vi "Dashboard Main.vi"() -> ()   [LabVIEW 2017]
uses:
  <vilib>/event_ctls.llb/eventvkey.ctl
  <vilib>/Rock Robotics/WPI/Dashboard/WPI_DashboardLogging Global.vi
  <vilib>/Utility/miscctls.llb/LVRowAndColumnTypeDef.ctl
  <vilib>/Rock Robotics/Network Tables/NT Write Boolean.vi
  <vilib>/Rock Robotics/Network Tables/NT Write Numeric Array.vi
  <vilib>/Rock Robotics/Network Tables/NT Read Numeric Array.vi
  <vilib>/Rock Robotics/Network Tables/NT Read Boolean Array.vi
panel:
  out "error out":errorcluster
  out "error out 2":errorcluster
  in  "Camera Settings Right":T1={"Frame Rate"=30, "Compression"=30, "Size"=1, "DB Camera Config"=FALSE} {"Frame Rate" scale=1.0..30.0; "Compression" scale=100.0..-1.0; "Size" items=["640x480", "320x240", "160x120"]}
  in  "Camera Name Right":string(combo)="No Camera Selection"
  out "Camera Info":cluster{"Mbps LED":bool, "Mbps":dbl, "fps":dbl} {"fps" format="%#.1g"; "Mbps" format="%#.1g"}
  in  "Camera Settings":T1={"Frame Rate"=30, "Compression"=30, "Size"=1, "DB Camera Config"=FALSE} {"Frame Rate" scale=1.0..30.0; "Compression" scale=100.0..-1.0; "Size" items=["640x480", "320x240", "160x120"]}
  in  "TCP":refnum<k5>
  in  "Rec Mode":enum32{"Stop", "Record", "Playback"}(radio)
  out "Robot IP":string
  out "Image Message":string="Timeout in Camera Communications"
  in  "Dashboard Tab":T2(tab)
  out "NT Connection":bool
  out "MotorChart R":cluster{"Numeric":dbl, "Numeric":dbl}(graph)
  out "MotorChart L":cluster{"Numeric":dbl, "Numeric":dbl}(graph)
  out "MotorSliders R":cluster{"MotorSlide1":dbl, "MotorSlide2":dbl} {"MotorSlide2" scale=-1.0..1.0 scale format="%#_2e"; "MotorSlide1" scale=-1.0..1.0 scale format="%#_2e"}
  out "MotorSliders L":cluster{"MotorSlide1":dbl, "MotorSlide2":dbl} {"MotorSlide2" scale=-1.0..1.0 scale format="%#_2e"; "MotorSlide1" scale=-1.0..1.0 scale format="%#_2e"}
  out "JS1 Z":dbl(slide) scale=-1.0..1.0 scale format="%#_2e"
  out "JS1 Graph":cluster{"X":dbl, "Y":dbl}[](graph)
  out "JS1 Buttons":T3
  out "JS2 Z":dbl(slide) scale=-1.0..1.0 scale format="%#_2e"
  out "JS2 Graph":cluster{"X":dbl, "Y":dbl}[](graph)
  out "JS2 Buttons":T3
  out "Mode":T4(ring)=enum."Auto Disabled"
  out "Gear State":string="Waiting...."
  out "Camera Image Right":T5(plugin-control)
  in  "Ring":u16(ring)
  in  "Select Robot Position":string(combo)="Select Robot Position ..."
  in  "Select Auto":string(combo)="Select Autonomous ..."
  in  "Left String":string
  in  "Right String":string
  in  "Save Left Auto":bool
  in  "Load Left Auto":bool
  in  "Save Right Auto":bool
  in  "Load Right Auto":bool
  out "new picture":picture
  in  "Starting Pos":i16(slide)=128 scale=340.0..50.0
  in  "Test Slider":dbl(slide) scale=0.0..100.0 scale format="%#_3g"
  in  "On/Off":bool caption="Solenoid"
  in  "Test Name":u16(ring) items=["Select the test to run..."]
  in  "Test Tree":string(tree)
  in  "Motor":cluster{"Value":dbl, "Enable":bool} {"Value" scale=-1.0..1.0 scale format="%#_3g"}
  out "Progress":T6 {"Test Progress" scale=0.0..100.0}
  in  "Rev/Fwd":cluster{"Forward":bool, "Reverse":bool}
  in  "Test Ring":u16(ring) items=["Monochrome", "Color"]
  out "Cmd Status":string
  in  "Execute Command":bool
  in  "Command Params":string[][](table)
  in  "Command Selection":i32(listbox)
  in  "CheckList":i32(listbox)
  out "Tree":string(tree)
  in  "Key Binds":u16[](array[ring]) items=["No Function", "Gear Shift", "Direction Toggle", "Cube Up", "Cube Down", "LRamp Deploy", "RRamp Deploy", "LRamp Raise", "RRamp Raise"]
  in  "High Gear":bool=TRUE
  in  "Direction Toggle":bool=TRUE
  in  "Autoshift":bool=TRUE
  in  "Max Speed":dbl=1.0 format="%#_13g"
  in  "Foreward Deadzone":dbl=1.0 format="%#_13g"
  in  "Turning Deadzone":dbl=0.4 format="%#_13g"
  in  "High Gear Turning Multiplier":dbl=0.65 format="%#_13g"
  in  "Save":bool
  in  "Load":bool
  out "Profile Name":string="Profile1"
  in  "Control System":T7(ring)
  in  "Turning Multiplier":dbl=1.0 format="%#_13g"
  out "Boolean Array":bool[](array[boolean])
  out "Time":dbl
  in  "Points Speed":dbl[][](array[slide]) scale=0.0..1.0
  out "Speed Graph":cluster{dbl[], dbl[]}[](graph)
  in  "Points Turning":dbl[][](array[slide]) scale=0.0..1.0
  out "Turning Graph":cluster{dbl[], dbl[]}[](graph)
  out "Camera Image":T5(plugin-control)
  out "Background":bool
  in  "Camera Name":string(combo)="No Camera Selection"
  # "HW"
  # "HW"
  # "Joysticks"
  # "Drive Motors"
  # "Front"
  # "Right"
  # "Left"
  # "Back"
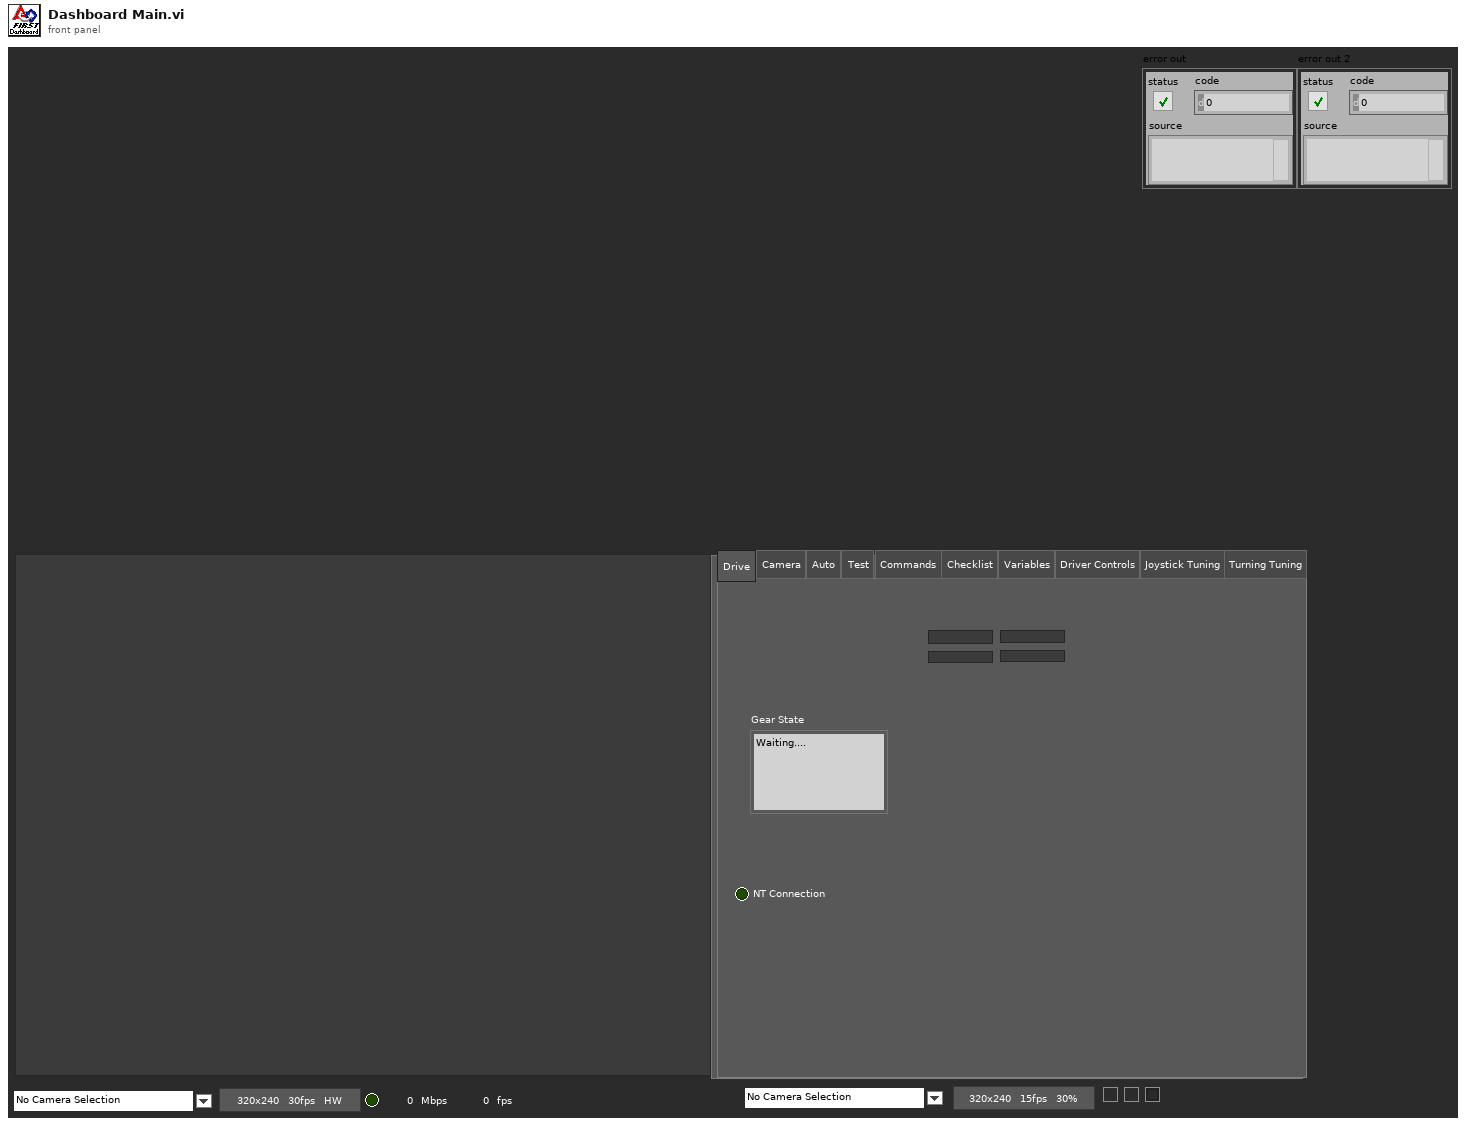
[diagram p1: front panel]
types:
  T1 = cluster{"Frame Rate":i32, "Compression":i32, "Size":u16, "DB Camera Config":bool}
  T2 = enum32{"Drive", "Camera", "Basic", "Auto", "Test", "Commands", "Checklist", "Variables", "Driver Controls", "Joystick Tuning", "Turning Tuning"}
  T3 = cluster{bool, bool, bool, bool, bool, bool, bool, bool, bool, bool, bool, bool}
  T4 = enum8{"Tele-Op Disabled", "Tele-Op Enabled", "Auto Disabled", "Auto Enabled", "Test Disabled", "Test Enabled", "Disconnected", "No Code", "E-Stop"}
  T5 = typedef "IMAQ Image.ctl" = refnum<image>
  T6 = cluster{"Test Progress":u8, "Test Progress Text":string}
  T7 = enum16{"Arcade Drive", "Two Part Arcade Drive", "Tank"}
  T8 = cluster{"Save Path":path, "Interval (s)":dbl, "Keep":i32}
  T9 = enum32{"Drive", "Camera", "Basic", "Custom", "Test", "Commands", "Checklist", "Variables"}
  T10 = typedef "Image Type" = u32
  T11 = cluster{"IDs":cluster{"RPC field ID":u16, "Unique ID":u16}, "String":string}
  T12 = enum32{"Drive", "Camera", "Basic", "Auto", "Test", "Commands", "Checklist", "Variables"}
  T13 = cluster{"Error Strings":string, "Disable Counts":cluster{u16, u16}, "Rail Faults":cluster{u16, u16, u16}, "Robot IP":string, "DB Mode":u8, "Event Info":cluster{"Name":string, "Type":u8, "Number":u16, "Replay":u8}}
  T14 = cluster{"Storage":cluster{"Disk Free":u64, "RAM Block":u32, "RAM free":u32}, "CPU Utilization":cluster{"CPU % ISR":sgl, "CPU % Time Crit":sgl, "CPU % Timed Str":sgl, "CPU % High":sgl, "CPU % Above":sgl, "CPU % Normal":sgl, "CPU % Low":sgl}, "CAN":cluster{"% Bus Utilization":sgl, "Bus Off Cnt":u32, "TX_FIFO Full Cnt":u32, "Receive Error Cnt":u8, "Transmit Error Cnt":u8}, "HID":cluster{"HID Outputs":u32, "Rumble Low":u16, "Rumble High":u16}[]}
  T15 = cluster{"Status bits":cluster{"Test Mode":bool, "Autonomous":bool, "Enabled":bool, "Code Start":bool, "Brownout":bool, "Reserved 2":bool, "Reserved 3":bool, "E-Stop":bool}, "Code Trace":cluster{"Disabled":bool, "TeleOp":bool, "Auto":bool, "Test":bool}, "Controller Type":enum16{"unknown", "cRIO", "roboRio"}, "Code?":enum16{"unknown", "noCode", "code"}, "Battery V":dbl}
  T16 = cluster{"Control Bits":cluster{"TestMode":bool, "Autonomous":bool, "Enabled":bool, "FMS Present":bool, bool, bool, bool, "E-Stop":bool}, "Team Station ":u8, "Countdown":sgl, "Joystick Values":cluster{"Axes":dbl[], "Buttons":bool[], "POVs":i16[]}[]}
  T17 = cluster{"Axes":dbl[], "Buttons":bool[], "POVs":i16[]}[]
  T18 = cluster{"Axes":dbl[], "Buttons":bool[], "POVs":i16[]}
  T19 = cluster{"Buttons[0]":bool, "Buttons[1]":bool, "Buttons[2]":bool, "Buttons[3]":bool, "Buttons[4]":bool, "Buttons[5]":bool, "Buttons[6]":bool, "Buttons[7]":bool, "Buttons[8]":bool, "Buttons[9]":bool, "Buttons[10]":bool, "Buttons[11]":bool}
  T20 = cluster{"High Gear Turning Multiplier":refnum<vi>, "Turning Deadzone":refnum<vi>, "Foreward Deadzone":refnum<vi>, "Max Speed":refnum<vi>, "Autoshift":refnum<vi>, "High Gear":refnum<vi>, "Direction Toggle":refnum<vi>, "Control System":refnum<vi>, "Turning Multiplier":refnum<vi>, "Profile Name":refnum<vi>, "Key Binds":refnum<vi>}
  T21 = cluster{"Camera Image":refnum<vi>, "Dashboard Tab":refnum<vi>, "Background":refnum<vi>, "Rec Mode":refnum<vi>, "Test Slider":refnum<vi>, "On/Off ":refnum<vi>, "Test Ring":refnum<vi>, "Rev/Fwd":refnum<vi>, "Test Name":refnum<vi>, "Motor":refnum<vi>, "Progress":refnum<vi>, "CheckList":refnum<vi>, "Tree":refnum<vi>, "Test Tree":refnum<vi>, "Command Params":refnum<vi>, "Command Selection":refnum<vi>, "Execute Command":refnum<vi>, "Cmd Status":refnum<vi>, "Camera Settings":refnum<vi>, "Camera Name":refnum<vi>, "Camera Info":refnum<vi>, "Camera Settings Right":refnum<vi>, "Camera Name Right":refnum<vi>, "Camera Image Right":refnum<vi>}
  T22 = cluster{"Camera Name Right":string, string, "Saved DB Images Info":cluster{"Save Path":path, "Interval (s)":dbl, "Keep":i32}}
  T23 = cluster{"Camera Name":string, string, "Saved DB Images Info":cluster{"Save Path":path, "Interval (s)":dbl, "Keep":i32}}
  T24 = cluster{"Operation":enum16{"Update", "Clear"}, "Color Box":u32}[]
  T25 = typedef "eventvkey.ctl" = enum16{"ASCII", "Enter", "Return", "Shift", "Ctrl", "Alt", "Cmd", "Opt", "Caps", "NumLock", "Clear", "Break", "Up", "Down", "Left", "Right", "Insert", "Delete", "Home", "End", "PageUp", "PageDown", "Escape", "Help", "Pause", "ScrollLock", "F1", "F2", "F3", "F4", "F5", "F6", "F7", "F8", "F9", "F10", "F11", "F12", "F13", "F14", "F15", "F16", "F17", "F18", "F19", "F20", "F21", "F22", "F23", "F24", "Play", "VolumeUp", "VolumeDown", "Mute", "Two Byte Char"}
  T26 = cluster{"Image Size":bool, "Image Type":bool, "Pixel Value":bool, "ROI Information":bool, "Zoom Factor":bool}
  T27 = cluster{"Operation":enum16{"Update", "Clear"}, "Color Box":u32}
  T28 = typedef "LVRowAndColumnTypeDef.ctl" = cluster{"Row":i32, "Column":i32}
  T29 = cluster{"Shift":bool, "Ctrl":bool, "Alt":bool, "Cmd":bool, "Opt":bool}
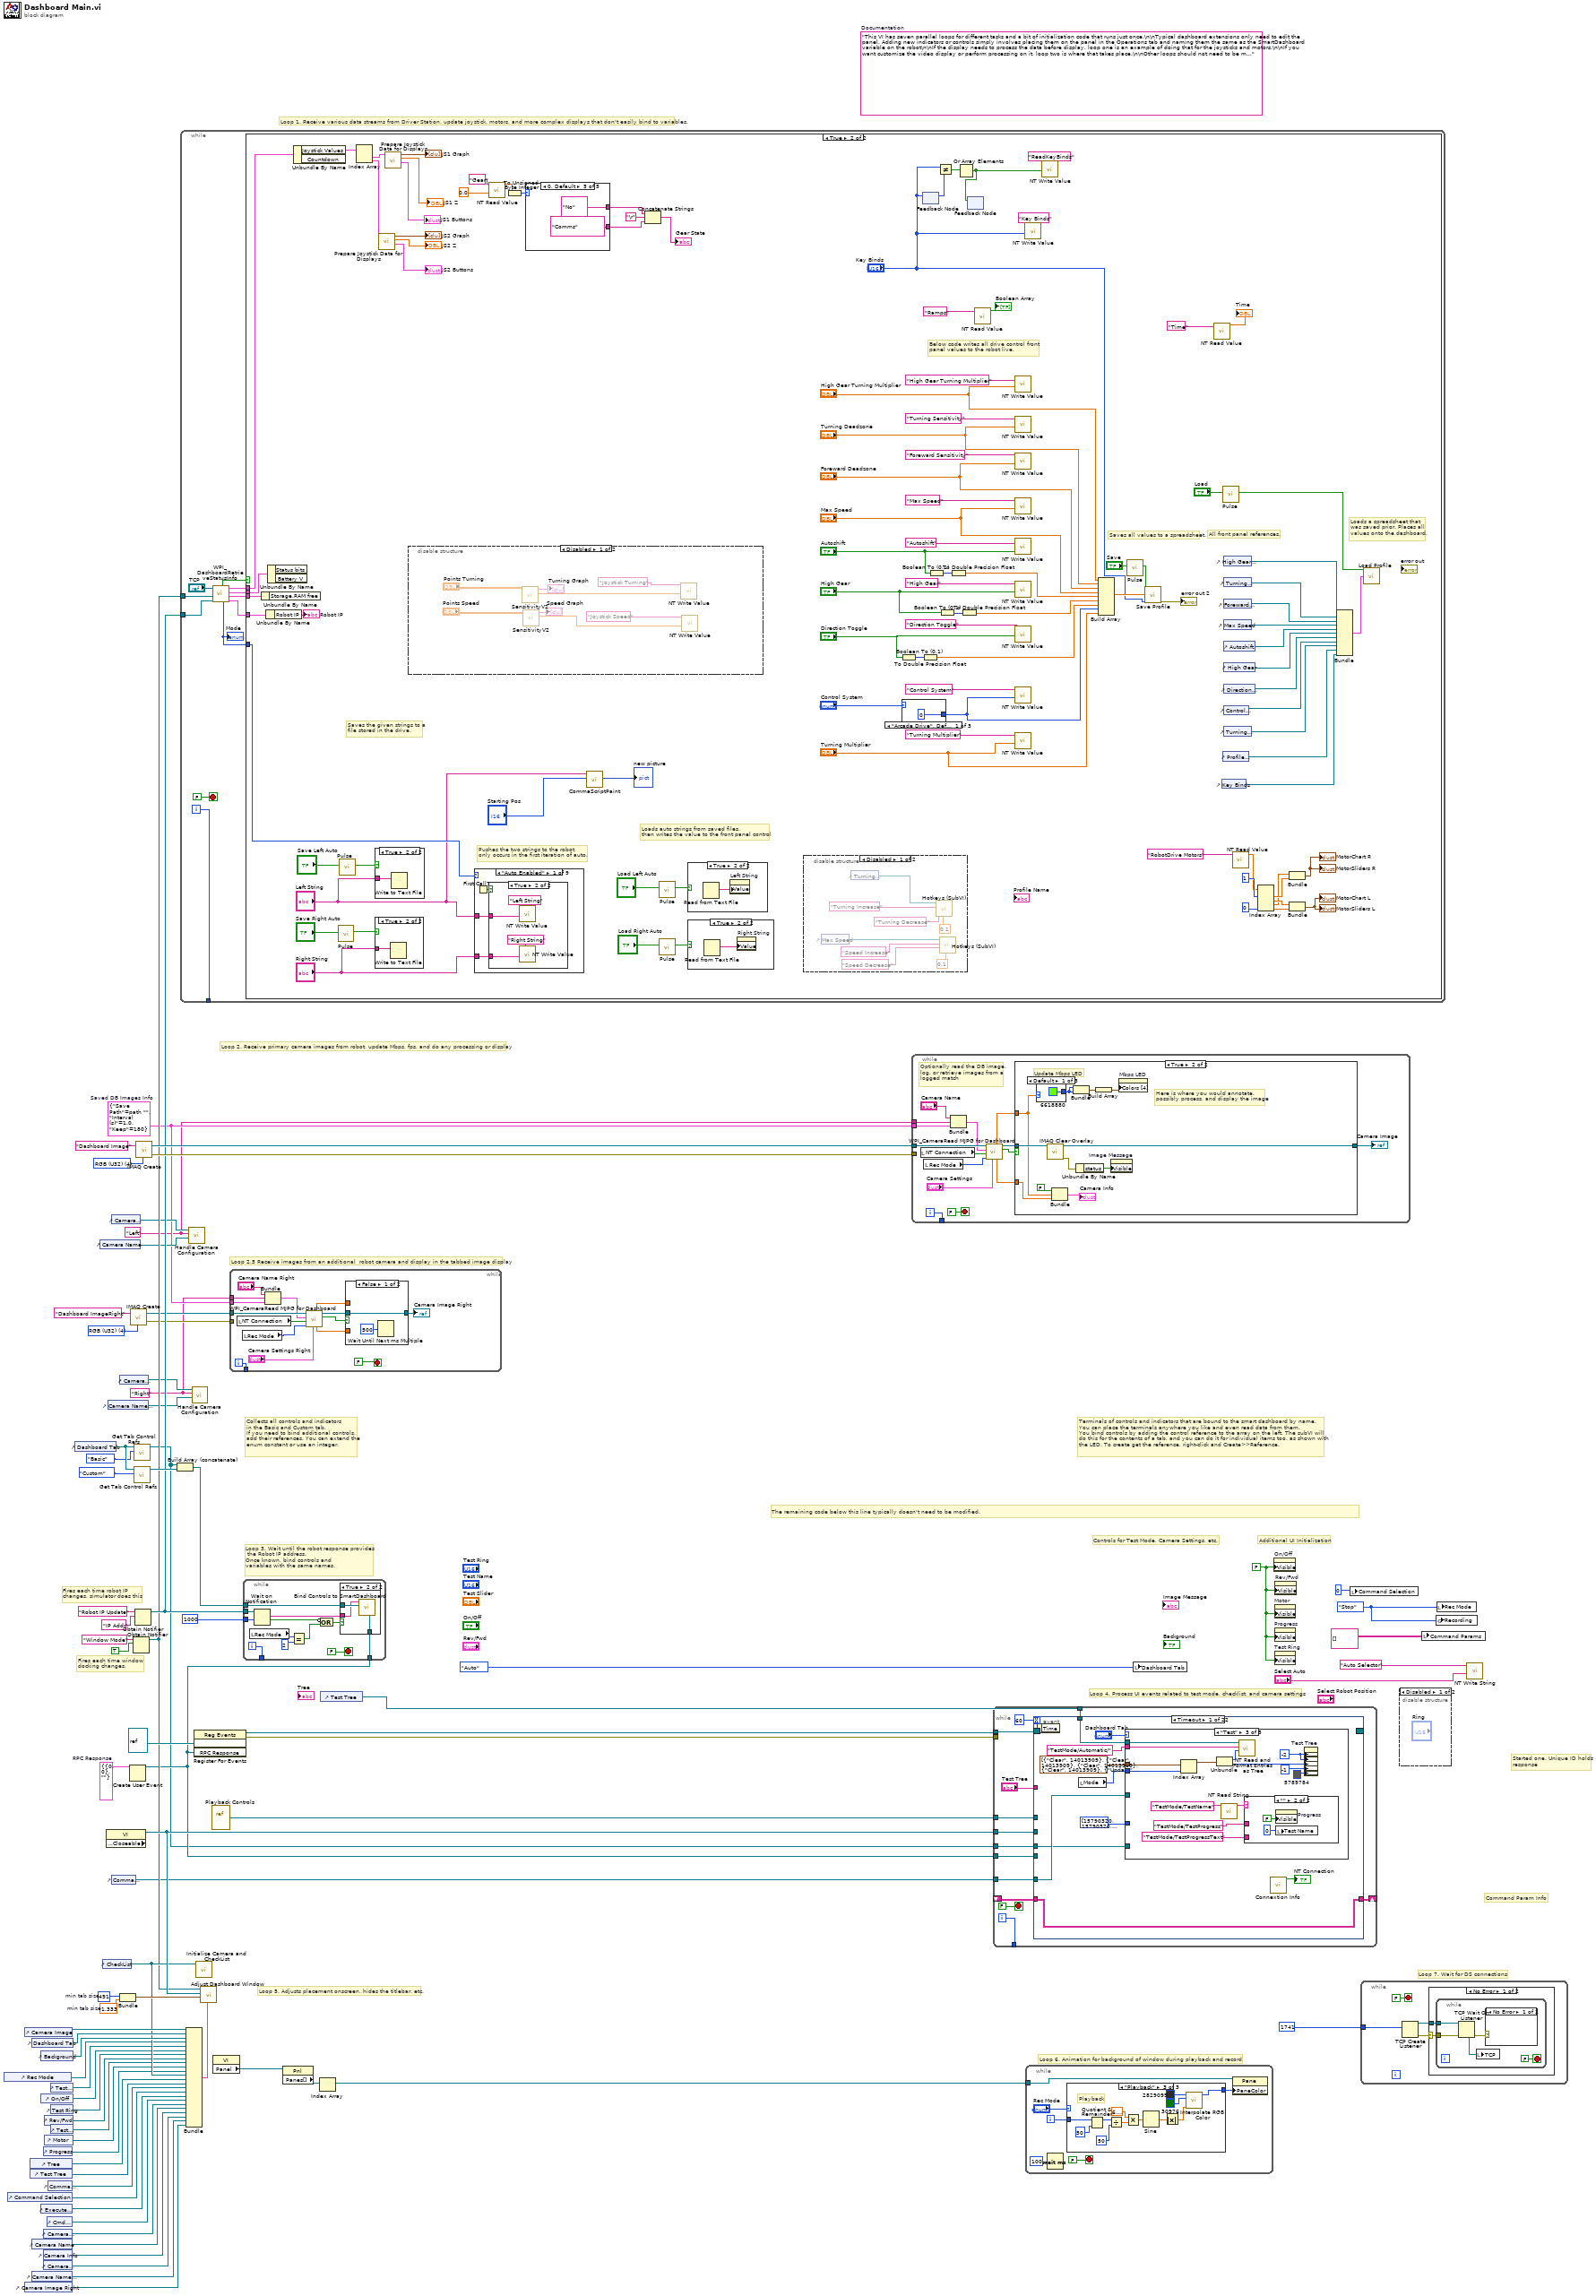
[diagram p0: block diagram]
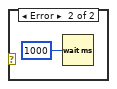
[diagram p4: hidden frame]
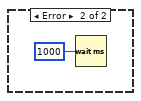
[diagram p5: hidden frame]
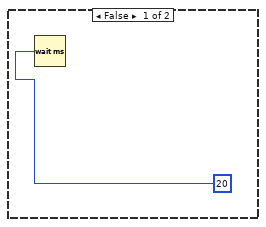
[diagram p6: hidden frame]
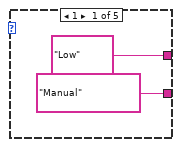
[diagram p8: hidden frame]
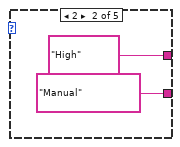
[diagram p9: hidden frame]
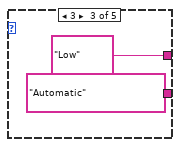
[diagram p10: hidden frame]
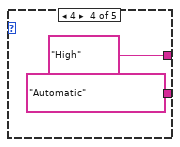
[diagram p11: hidden frame]
diagram:
  w4 = T8 {"Save Path"=path "", "Interval (s)"=1.0, "Keep"=180}  # Saved DB Images Info
  w3 = "Right"
  w2 = "Left"
  w14 = T10 4 items=["Grayscale (U8)", "Grayscale (I16)", "Grayscale (SGL)", "Complex (CSG)", "RGB (U32)", "HSL (U32)", "RGB (U64)"] ("Image Type")
  w29 = T11 {"IDs"={"RPC field ID"=0, "Unique ID"=0}, "String"=""}  # RPC Response
  w52 = 491  # min tab size
  w51 = 1.333  # min tab size
  w59 = enum32{"Stop", "Record", "Playback"}."Stop" ("Rec Mode")
  w36 = FALSE ("Visible")
  (unwired) "This VI has seven parallel loops for different tasks and a bit of initialization code that runs just once.\n\nTypical dashboard extensions only need to edit the panel. Adding new indicators or controls simply involves placing them on the panel in the Operations tab and naming them the same as the SmartDashboard variable on the robot\n\nIf the display needs to process the data before display, loop one is an example of doing that for the joysticks and motors.\n\nIf you want customize the video display or perform processing on it, loop two is where that takes place.\n\nOther loops should not need to be modified. They are pretty standard, and document the task they perform."  # Documentation
  w76 = T10 4 items=["Grayscale (U8)", "Grayscale (I16)", "Grayscale (SGL)", "Complex (CSG)", "RGB (U32)", "HSL (U32)", "RGB (U64)"] ("Image Type")
  # "Loop 2.5 Receive images from an additional  robot camera and display in the tabbed image display"
  # "Command Param Info"
  # "Started one, Unique ID holds\nresponse"
  # "Loop 7. Wait for DS connections"
  # "Controls for Test Mode, Camera Settings, etc."
  # "Additional UI Initialization"
  # "Loop 6. Animation for background of window during playback and record"
  # "Fires each time robot IP\nchanges, simulator does this"
  # "Fires each time window\ndocking changes."
  # "Collects all controls and indicators\nin the Basic and Custom tab.\nIf you need to bind additional controls,\nadd their references. You can extend the\nenum constant or use an integer."
  # "The remaining code below this line typically doesn't need to be modified."
  # "Loop 4. Process UI events related to test mode, checklist, and camera settings"
  # "Terminals of controls and indicators that are bound to the smart dashboard by name.\nYou can place the terminals anywhere you like and even read data from them.\nYou bind controls by adding the control reference to the array on the left. The subVI will\ndo this for the contents of a tab, and you can do it for individual items too, as shown with\nthe LED. To create get the reference, right-click and Create>>Reference."
  # "Loop 3. Wait until the robot response provides\n the Robot IP address.\nOnce known, bind controls and\nvariables with the same names."
  # "Loop 5. Adjusts placement onscreen, hides the titlebar, etc."
  # "Loop 1. Receive various data streams from Driver Station, update joystick, motors, and more complex displays that don't easily bind to variables."
  # "Loop 2. Receive primary camera images from robot, update Mbps, fps, and do any processing or display"
  n1 = control-ref of="Rec Mode"() -> (w42:refnum<vi>)
  n2 = control-ref of="Command Selection"() -> (w28:refnum<vi>)
  n3 = control-ref of="Camera Image Right"() -> (w7:refnum<vi>)
  n4 = control-ref of="Camera Image"() -> (w54:refnum<vi>)
  n5 = control-ref of="Tree"() -> (w46:refnum<vi>)
  n6 = control-ref of="Test Tree"() -> (w45:refnum<vi>)
  n7 = control-ref of="Dashboard Tab"() -> (w53:refnum<vi>)
  n8 = control-ref of="Camera Name"() -> (w19:refnum<vi>)
  n9 = control-ref of="Camera Name Right"() -> (w8:refnum<vi>)
  n10 = control-ref of="Execute Command"() -> (w30:refnum<vi>)
  n11 = control-ref of="Background"() -> (w49:refnum<vi>)
  n12 = control-ref of="On/Off"() -> (w40:refnum<vi>)
  n13 = control-ref of="Progress"() -> (w37:refnum<vi>)
  n14 = control-ref of="Camera Settings"() -> (w20:refnum<vi>)
  n15 = control-ref of="Camera Info"() -> (w18:refnum<vi>)
  n16 = control-ref of="Camera Settings Right"() -> (w9:refnum<vi>)
  n17 = control-ref of="Rev/Fwd"() -> (w38:refnum<vi>)
  n18 = control-ref of="Motor"() -> (w43:refnum<vi>)
  n19 = control-ref of="Cmd Status"() -> (w24:refnum<vi>)
  n20 = control-ref of="Command Params"() -> (w31:refnum<vi>)
  n21 = control-ref of="Test Slider"() -> (w41:refnum<vi>)
  n22 = control-ref of="Test Ring"() -> (w39:refnum<vi>)
  n23 = control-ref of="Test Name"() -> (w44:refnum<vi>)
  n24 = control-ref of="Dashboard Tab"() -> (w57:refnum<vi>)
  n25 = control-ref of="Camera Name"() -> (w21:refnum<vi>)
  n26 = control-ref of="CheckList"() -> (w47:refnum<vi>)
  n27 = property class="VI" props=["Front Panel.Closeable"]() -> (reference out=w58:refnum<vi>)  [unwired: 2 in, 2 out]
  n28 = control-ref of="Camera Name Right"() -> (w10:refnum<vi>)
  n29 = control-ref of="Camera Settings"() -> (w22:refnum<vi>)
  n30 = control-ref of="Command Params"() -> (w23:refnum<vi>)
  n31 = control-ref of="Camera Settings Right"() -> (w11:refnum<vi>)
  n32 = Bundle("min tab size"=w52, "min tab size"=w51) -> (w50:cluster{"min tab size":i32, "min tab size":dbl})  [unwired: 1 in]
  n33 = Create User Event(user event datatype=w29) -> (user event=w25:refnum<user-event>)  [unwired: 1 in, 1 out]
  n34 = call "IMAQ Create"("Image Name"="Dashboard ImageRight", "Image Type"=w14) -> ("New Image"=w13:T5, "error out"=w12:errorcluster)  [unwired: 2 in, 1 out]
  n35 = Obtain Notifier(name (unnamed)="Window Mode", notification data type=TRUE) -> (notifier out=w34:refnum<notifier>)  [unwired: 2 in, 2 out]
  n36 = call <vilib>:"Get Tab Control Refs.vi"("Page Index"=T9."Basic" ("Dashboard Tab"), "TabControl in"=w57) -> ("ControlsOnPage"=w17:refnum<vi>[])  [unwired: 9 in]
  n37 = call <vilib>:"Get Tab Control Refs.vi"("Page Index"=T9."Custom" ("Dashboard Tab"), "TabControl in"=w57) -> ("ControlsOnPage"=w56:refnum<vi>[])  [unwired: 9 in]
  n38 = Obtain Notifier(name (unnamed)="Robot IP Update", notification data type="IP Addr" ("name (unnamed)")) -> (notifier out=w35:refnum<notifier>)  [unwired: 2 in, 2 out]
  n39 = call "IMAQ Create"("Image Name"="Dashboard Image", "Image Type"=w76) -> ("New Image"=w74:T5, "error out"=w73:errorcluster)  [unwired: 2 in, 1 out]
  n40 = Build Array (concatenate)(w17, w56) -> (w55:refnum<vi>[])
  n41 = while {
    tunnel: [w86] -> _
    tunnel: w35 -> [w80]
    tunnel: w34 -> [w77]
    i -> [w86]
    stop <- FALSE stop-if-true
    n42 = call <vilib>:"WPI_DashboardRetrieveStatusInfo.vi"("Binding Refnum"=w80, "Window Mode Notifier"=w77, "TCP Cnx"="TCP") -> ("Power and Errors"=w81:T13, "Robot Metrics"=w84:T14, "Status Info"=w85:T15, "Control Info"=w82:T16, "Robot Mode"=w79:T4, "Process?"=w83:bool)  [unwired: 3 in]
    "Mode" <- w79
    n43 = case shown="True" w83 {
      tunnel: w85 -> [_ w186]
      tunnel: w84 -> [_ w185]
      tunnel: w82 -> [_ w184]
      tunnel: w81 -> [_ w183]
      tunnel: w79 -> [_ w113]
      frame False {
        n44 = Wait (ms)(milliseconds to wait=u32 20) -> ()  [unwired: 1 out]
      }
      frame True {
        # "Loads a spreadsheet that\nwas saved prior. Places all\nvalues onto the dashboard."
        # "All front panel references."
        # "Saves all values to a spreadsheet."
        # "Below code writes all drive control front\npanel values to the robot live."
        # "Pushes the two strings to the robot,\nonly occurs in the first iteration of auto."
        # "Saves the given strings to a\nfile stored in the drive."
        # "Loads auto strings from saved files,\nthen writes the value to the front panel control"
        n45 = Unbundle By Name(w185) -> ()  [unwired: 1 out]
        n46 = Unbundle By Name(w183) -> ("Robot IP"=→"Robot IP":string)
        n47 = Unbundle By Name(w186) -> ()  [unwired: 2 out]
        n48 = Unbundle By Name(w184) -> ("Joystick Values"=w174:T17)  [unwired: 1 out]
        n49 = call "Pulse.vi"("Input"="Save Right Auto") -> ("Output"=w117:bool)  [unwired: 10 in]
        n50 = call "Pulse.vi"("Input"="Save Left Auto") -> ("Output"=w121:bool)  [unwired: 10 in]
        n51 = Index Array(array=w174) -> (element #1=w173:T18, element #2=w169:T18)  [unwired: 2 in]
        n52 = case shown="True" w117 {
          tunnel: "Right String" -> [_ w220]
          frame False {
          }
          frame True {
            n53 = Write to Text File(text=w220) -> ()  [unwired: 3 in, 3 out]
          }
        }
        n54 = case shown="True" w121 {
          tunnel: "Left String" -> [_ w223]
          frame False {
          }
          frame True {
            n55 = Write to Text File(text=w223) -> ()  [unwired: 3 in, 3 out]
          }
        }
        n56 = call "Prepare Joystick Data for Displays.vi"("Joystick Values"=w169) -> ("Buttons"=→"JS2 Buttons":T19, "Z Axis"=→"JS2 Z":dbl, "Cartesian Data"=→"JS2 Graph":cluster{"X axis":dbl, "X axis":dbl}[])  [unwired: 8 in]
        n57 = call "Prepare Joystick Data for Displays.vi"("Joystick Values"=w173) -> ("Buttons"=→"JS1 Buttons":T19, "Z Axis"=→"JS1 Z":dbl, "Cartesian Data"=→"JS1 Graph":cluster{"X axis":dbl, "X axis":dbl}[])  [unwired: 8 in]
        n58 = disable-structure shown="Disabled" {
          frame Disabled {
            n59 = call "SensitivityV2.vi"("Points"="Points Turning") -> ("Yi"=w187:dbl[], "XY Graph"=→"Turning Graph":cluster{dbl[], dbl[]}[])  [unwired: 9 in]
            n60 = call "SensitivityV2.vi"("Points"="Points Speed") -> ("Yi"=w190:dbl[], "XY Graph"=→"Speed Graph":cluster{dbl[], dbl[]}[])  [unwired: 9 in]
            n61 = call-poly <vilib>:"NT Write Value.vi"("Numeric Array"=w187, "Name"="Joystick Turning") -> ()  [unwired: 9 in, 1 out]
            n62 = call-poly <vilib>:"NT Write Value.vi"("Numeric Array"=w190, "Name"="Joystick Speed") -> ()  [unwired: 9 in, 1 out]
          }
          frame Enabled {
          }
        }
        n63 = case shown="\"Auto Enabled\"" w113 {
          tunnel: "Left String" -> [w215 _ _ _ _ _ _ _ _]
          tunnel: "Right String" -> [w214 _ _ _ _ _ _ _ _]
          frame "Auto Enabled" {
            n64 = First Call?() -> (First Call?: T/F=w213:bool)
            n65 = case shown="True" w213 {
              tunnel: w215 -> [_ w219]
              tunnel: w214 -> [_ w218]
              frame False {
              }
              frame True {
                n66 = call-poly <vilib>:"NT Write Value.vi"("String"=w219, "Name"="Left String") -> ()  [unwired: 9 in, 1 out]
                n67 = call-poly <vilib>:"NT Write Value.vi"("String"=w218, "Name"="Right String") -> ()  [unwired: 9 in, 1 out]
              }
            }
          }
          frame "Test Disabled" {
          }
          frame "Test Enabled" {
          }
          frame "Disconnected" {
          }
          frame "No Code" {
          }
          frame "E-Stop" {
          }
          frame "Auto Disabled" {
          }
          frame "Tele-Op Enabled" {
          }
          frame "Tele-Op Disabled" {
          }
        }
        n68 = call-poly <vilib>:"NT Read Value.vi"("Default Value"=0.0, "Name"="Gear") -> ("Numeric"=w106:dbl)  [unwired: 8 in, 1 out]
        n69 = To Unsigned Byte Integer(number=w106) -> (unsigned 8bit integer=w105:u8)
        n70 = case shown="0, Default" w105 {
          tunnel: ["Low" "High" "Low" "High" "No"] -> w109
          tunnel: ["Manual" "Manual" "Automatic" "Automatic" "Comms"] -> w111
          frame 1 {
          }
          frame 2 {
          }
          frame 3 {
          }
          frame 4 {
          }
          frame 0, Default {
          }
        }
        n71 = call "CommaScriptPaint.vi"("string 2"="Starting Pos", "string"="Left String") -> ("new picture"=→"new picture":picture)  [unwired: 8 in, 1 out]
        n72 = Concatenate Strings(w109, "\r", w111) -> (→"Gear State":string)
        n73 = call "Pulse.vi"("Input"="Load Left Auto") -> ("Output"=w120:bool)  [unwired: 10 in]
        n74 = call "Pulse.vi"("Input"="Load Right Auto") -> ("Output"=w114:bool)  [unwired: 10 in]
        n75 = case shown="True" w120 {
          frame False {
          }
          frame True {
            n76 = Read from Text File() -> (text=w222:string)  [unwired: 4 in, 3 out]
            n77 = property on="Left String" class="Str"("Value"=w222) -> ()  [unwired: 2 in, 2 out]
          }
        }
        n78 = case shown="True" w114 {
          frame False {
          }
          frame True {
            n79 = Read from Text File() -> (text=w221:string)  [unwired: 4 in, 3 out]
            n80 = property on="Right String" class="Str"("Value"=w221) -> ()  [unwired: 2 in, 2 out]
          }
        }
        n81 = disable-structure shown="Disabled" {
          frame Disabled {
            n82 = control-ref of="Max Speed"() -> (w209:refnum<vi>)
            n83 = control-ref of="Turning Multiplier"() -> (w212:refnum<vi>)
            n84 = call "Hotkeys (SubVI).vi"("Iteration Quantity"=0.1, "Decrease"="Turning Decrease", "Increase"="Turning Increase", "Reference"=w212) -> ()  [unwired: 8 in]
            n85 = call "Hotkeys (SubVI).vi"("Iteration Quantity"=0.1, "Decrease"="Speed Decrease", "Increase"="Speed Increase", "Reference"=w209) -> ()  [unwired: 8 in]
          }
          frame Enabled {
          }
        }
        n86 = Boolean To (0,1)(Boolean="Direction Toggle") -> (0, 1=w145:i16)
        n87 = case shown="\"Arcade Drive\", Default" "Control System" {
          tunnel: [0 1 2] -> w122
          frame "Arcade Drive", Default {
          }
          frame "Two Part Arcade Drive" {
          }
          frame "Tank" {
          }
        }
        n88 = feedback-in #1("Key Binds") -> ()
        n89 = feedback #1() -> (w104:u16[])  [unwired: 1 in]
        n90 = To Double Precision Float(number=w145) -> (double precision float=w146:dbl)
        n91 = Boolean To (0,1)(Boolean="Autoshift") -> (0, 1=w141:i16)
        n92 = Not Equal?(x="Key Binds", y=w104) -> (x != y?=w103:bool[])
        n93 = Boolean To (0,1)(Boolean="High Gear") -> (0, 1=w143:i16)
        n94 = To Double Precision Float(number=w141) -> (double precision float=w142:dbl)
        n95 = Or Array Elements(Boolean array=w103) -> (logical OR=w101:bool)
        n96 = To Double Precision Float(number=w143) -> (double precision float=w144:dbl)
        n97 = feedback-in #2(w101) -> ()
        n98 = feedback #2() -> ()  [unwired: 2 in]
        n99 = call-poly <vilib>:"NT Read Value.vi"("Name"="Ramps") -> ("Boolean Array"=→"Boolean Array":bool[])  [unwired: 9 in, 1 out]
        n100 = call-poly <vilib>:"NT Write Value.vi"("Numeric"="High Gear Turning Multiplier", "Name"="High Gear Turning Multiplier") -> ()  [unwired: 9 in, 1 out]
        n101 = call-poly <vilib>:"NT Write Value.vi"("Numeric"="Turning Deadzone", "Name"="Turning Sensitivity") -> ()  [unwired: 9 in, 1 out]
        n102 = call-poly <vilib>:"NT Write Value.vi"("Numeric"="Foreward Deadzone", "Name"="Foreward Sensitivity") -> ()  [unwired: 9 in, 1 out]
        n103 = call-poly <vilib>:"NT Write Value.vi"("Numeric"="Max Speed", "Name"="Max Speed") -> ()  [unwired: 9 in, 1 out]
        n104 = call-poly <vilib>:"NT Write Value.vi"("Boolean"="Autoshift", "Name"="Autoshift") -> ()  [unwired: 9 in, 1 out]
        n105 = call-poly <vilib>:"NT Write Value.vi"("Boolean"="High Gear", "Name"="High Gear") -> ()  [unwired: 9 in, 1 out]
        n106 = call-poly <vilib>:"NT Write Value.vi"("Boolean"="Direction Toggle", "Name"="Direction Toggle") -> ()  [unwired: 9 in, 1 out]
        n107 = call-poly <vilib>:"NT Write Value.vi"("Numeric"=w122, "Name"="Control System") -> ()  [unwired: 9 in, 1 out]
        n108 = call-poly <vilib>:"NT Write Value.vi"("Numeric"="Turning Multiplier", "Name"="Turning Multiplier") -> ()  [unwired: 9 in, 1 out]
        n109 = call-poly <vilib>:"NT Write Value.vi"("Numeric Array"="Key Binds", "Name"="Key Binds") -> ()  [unwired: 9 in, 1 out]
        n110 = call-poly <vilib>:"NT Write Value.vi"("Boolean"=w101, "Name"="ReadKeyBinds") -> ()  [unwired: 9 in, 1 out]
        n111 = Build Array("High Gear Turning Multiplier", "Turning Deadzone", "Foreward Deadzone", "Max Speed", w142, w144, w146, w122, "Turning Multiplier") -> (w148:dbl[])
        n112 = call "Pulse.vi"("Input"="Save") -> ("Output"=w140:bool)  [unwired: 10 in]
        n113 = call "Save Profile.vi"("Key Binds"="Key Binds", "Driver Pref"=w148, "Output"=w140) -> ("error out"=→"error out 2":errorcluster)  [unwired: 8 in]
        n114 = call-poly <vilib>:"NT Read Value.vi"("Name"="Time") -> ("Numeric"=→"Time":dbl)  [unwired: 9 in, 1 out]
        n115 = control-ref of="Key Binds"() -> (w98:refnum<vi>)
        n116 = call "Pulse.vi"("Input"="Load") -> ("Output"=w137:bool)  [unwired: 10 in]
        n117 = control-ref of="Profile Name"() -> (w125:refnum<vi>)
        n118 = control-ref of="High Gear Turning Multiplier"() -> (w136:refnum<vi>)
        n119 = control-ref of="Turning Deadzone"() -> (w135:refnum<vi>)
        n120 = control-ref of="Foreward Deadzone"() -> (w134:refnum<vi>)
        n121 = control-ref of="Max Speed"() -> (w133:refnum<vi>)
        n122 = control-ref of="Autoshift"() -> (w132:refnum<vi>)
        n123 = control-ref of="High Gear"() -> (w131:refnum<vi>)
        n124 = control-ref of="Direction Toggle"() -> (w130:refnum<vi>)
        n125 = control-ref of="Control System"() -> (w128:refnum<vi>)
        n126 = control-ref of="Turning Multiplier"() -> (w124:refnum<vi>)
        n127 = call-poly <vilib>:"NT Read Value.vi"("Name"="RobotDrive Motors") -> ("Numeric Array"=w164:dbl[])  [unwired: 9 in, 1 out]
        n128 = Index Array(array=w164, index #1=1, index #4=0) -> (element #1=w178:dbl, element #2=w179:dbl, element #3=w177:dbl, element #4=w182:dbl)  [unwired: 2 in]
        n129 = Bundle("Numeric"=w177, "Numeric"=w178) -> (→"MotorChart R" →"MotorSliders R":cluster{"Numeric":dbl, "Numeric":dbl})  [unwired: 1 in]
        n130 = Bundle("Numeric"=w179, "Numeric"=w182) -> (→"MotorChart L" →"MotorSliders L":cluster{"Numeric":dbl, "Numeric":dbl})  [unwired: 1 in]
        n131 = Bundle("High Gear Turning Multiplier"=w136, "Turning Deadzone"=w135, "Foreward Deadzone"=w134, "Max Speed"=w133, "Autoshift"=w132, "High Gear"=w131, "Direction Toggle"=w130, "Control System"=w128, "Turning Multiplier"=w124, "Profile Name"=w125, "Key Binds"=w98) -> (w97:T20)  [unwired: 1 in]
        n132 = call "Load Profile.vi"("Output"=w137, "References"=w97) -> ()  [unwired: 14 in]
      }
    }
  }
  n133 = Bundle("Camera Image"=w54, "Dashboard Tab"=w53, "Background"=w49, "Rec Mode"=w42, "Test Slider"=w41, "On/Off"=w40, "Test Ring"=w39, "Rev/Fwd"=w38, "Test Name"=w44, "Motor"=w43, "Progress"=w37, "CheckList"=w47, "Tree"=w46, "Test Tree"=w45, "Command Params"=w31, "Command Selection"=w28, "Execute Command"=w30, "Cmd Status"=w24, "Camera Settings"=w20, "Camera Name"=w19, "Camera Info"=w18, "Camera Settings Right"=w9, "Camera Name Right"=w8, "Camera Image Right"=w7) -> (w48:T21)  [unwired: 1 in]
  n134 = call "Handle Camera Configuration.vi"("CameraNameRef"=w21, "Display Name"=w2, "ClusterRef"=w22) -> ()  [unwired: 9 in]
  n135 = call "Handle Camera Configuration.vi"("CameraNameRef"=w10, "Display Name"=w3, "ClusterRef"=w11) -> ()  [unwired: 9 in]
  n136 = register-events(refnum<vi> refnum, w25) -> (reference out=w63:refnum<event-registration>, error out=w62:errorcluster)  [unwired: 2 in]
  n137 = call "Initialize Camera and CheckList.vi"("ListBox in"=w47) -> ()  [unwired: 11 in]
  n138 = call "Adjust Dashboard Window.vi"("Sizing Refnums"=w48, "Size Constraints"=w50, "VI"=w58, "WIn Mode"=w34) -> ()  [unwired: 8 in]
  n139 = vi-ref "Playback Controls.vi"() -> (w64:refnum<vi>)
  n140 = property class="VI"() -> ("Panel"=w66:refnum<vi>)  [unwired: 2 in, 2 out]
  n141 = while {
    tunnel: w13 -> [w241]
    tunnel: w12 -> [_]
    tunnel: [w236] -> _
    tunnel: w4 -> [w230]
    tunnel: w3 -> [w227]
    i -> [w236]
    stop <- FALSE stop-if-true
    n142 = local read "NT Connection"() -> (w231:bool)
    n143 = local read "Rec Mode"() -> (w240:enum32{"Stop", "Record", "Playback"})
    n144 = Bundle("Camera Name Right"="Camera Name Right", w227, "Saved DB Images Info"=w230) -> (w229:T22)  [unwired: 1 in]
    n145 = call <vilib>:"WPI_CameraRead MJPG for Dashboard.vi"("Camera Settings"="Camera Settings Right", "Rec Mode"=w240, "NT Connection"=w231, "Capture Info"=w229, "Refnum in"=w241) -> ("Active"=w235:bool, "Refnum out"=w238:T5, "FPS"=w233:dbl, "Bandwidth (Mbps)"=w234:dbl)  [unwired: 3 in]
    n146 = case shown="False" w235 {
      tunnel: w238 -> [w242 w244]
      tunnel: w234 -> [_ _]
      tunnel: w233 -> [_ _]
      tunnel: [w242 w244] -> w232
      frame False {
        n147 = Wait Until Next ms Multiple(millisecond multiple=u32 500) -> ()  [unwired: 1 out]
      }
      frame True {
      }
    }
    "Camera Image Right" <- w232
  }
  n148 = while {
    tunnel: w55 -> [w256]
    tunnel: w35 -> [w254]
    tunnel: [w252] -> _
    tunnel: u32 1000 ("milliseconds to wait") -> [w251]
    tunnel: w25 -> [w245]
    i -> [w252]
    stop <- FALSE stop-if-true
    n149 = local read "Rec Mode"() -> (w247:enum32{"Stop", "Record", "Playback"})
    n150 = Wait on Notification(notifier=w254, timeout in ms (-1)=w251) -> (notification=w253:string, timed out?=w249:bool)  [unwired: 2 in, 2 out]
    n151 = Equal?(x=w247, y=u16 2 ("Rec Mode")) -> (x = y?=w248:bool)
    n152 = Compound Arithmetic op=OR(invert w249, w248) -> (w250:bool)
    n153 = case shown="True" w250 {
      tunnel: w256 -> [_ w259]
      tunnel: w253 -> [_ w258]
      tunnel: w245 -> [_ w257]
      frame False {
      }
      frame True {
        n154 = call <vilib>:"Bind Controls to SmartDashboard.vi"("RPC ref"=w257, "Bound Control Refs"=w259, "Server IP Address"=w258) -> ()  [unwired: 9 in]
      }
    }
  }
  n155 = property class="Pnl"(reference=w66) -> ("Panes[]"=w67:refnum<vi>[])  [unwired: 1 in, 2 out]
  n156 = Index Array(array=w67) -> (element=w65:refnum<vi>)  [unwired: 1 in]
  n157 = control-ref of="Test Tree"() -> (w68:refnum<vi>)
  n158 = while {
    tunnel: w74 -> [w272]
    tunnel: w73 -> [_]
    tunnel: [w273] -> _
    tunnel: w4 -> [w263]
    tunnel: w2 -> [w260]
    i -> [w273]
    stop <- FALSE stop-if-true
    # "Optionally read the DB image,\nlog, or retrieve images from a\nlogged match"
    n159 = local read "NT Connection"() -> (w264:bool)
    n160 = local read "Rec Mode"() -> (w268:enum32{"Stop", "Record", "Playback"})
    n161 = Bundle("Camera Name"="Camera Name", w260, "Saved DB Images Info"=w263) -> (w262:T23)  [unwired: 1 in]
    n162 = call <vilib>:"WPI_CameraRead MJPG for Dashboard.vi"("Camera Settings"="Camera Settings", "Rec Mode"=w268, "NT Connection"=w264, "Capture Info"=w262, "Refnum in"=w272) -> ("Active"=w270:bool, "Refnum out"=w271:T5, "FPS"=w269:dbl, "Bandwidth (Mbps)"=w267:dbl)  [unwired: 3 in]
    n163 = case shown="True" w270 {
      tunnel: w271 -> [w275 w286]
      tunnel: w267 -> [_ w283]
      tunnel: w269 -> [_ w284]
      tunnel: [w275 w280] -> w265
      frame False {
        w277 = u32 1985280 ("Color Box")
        # "Sleep for 500ms"
        n164 = Bundle("Color Box"=w277, "Color Box"=w277) -> (w278:cluster{"Color Box":u32, "Color Box":u32})  [unwired: 1 out]
        n165 = Build Array(w278) -> (w276:cluster{"Color Box":u32, "Color Box":u32}[])
        n166 = property on="Mbps LED" class="Bool (strict)"("Colors [4]"=w276) -> ()  [unwired: 2 in, 2 out]
        n167 = Wait Until Next ms Multiple(millisecond multiple=u32 500) -> ()  [unwired: 1 out]
      }
      frame True {
        # "Here is where you would annotate,\npossibly process, and display the image"
        # "Update Mbps LED"
        n168 = case shown="Default" w283 {
          tunnel: [u32 6618880 ("Color Box") u32 16776722 ("Color Box") u32 16716800 ("Color Box")] -> w287
          frame Default {
          }
          frame 4, 5 {
          }
          frame 6.. {
          }
        }
        n169 = call "IMAQ Clear Overlay"("Image"=w286) -> ("error out"=w289:errorcluster, "Image Out"=w280:T5)  [unwired: 2 in, 7 out]
        n170 = Bundle(FALSE, "Bandwidth (Mbps)"=w283, "FPS"=w284) -> (→"Camera Info":cluster{bool, "Bandwidth (Mbps)":dbl, "FPS":dbl})  [unwired: 1 in]
        n171 = Bundle("Color Box"=w287, "Color Box"=w287) -> (w288:cluster{"Color Box":u32, "Color Box":u32})  [unwired: 1 out]
        n172 = Unbundle By Name(w289) -> ("status"=w290:bool)
        n173 = Build Array(w288) -> (w285:cluster{"Color Box":u32, "Color Box":u32}[])
        n174 = property on="Image Message" class="Str"("Visible"=w290) -> ()  [unwired: 2 in, 2 out]
        n175 = property on="Mbps LED" class="Bool (strict)"("Colors [4]"=w285) -> ()  [unwired: 2 in, 2 out]
      }
    }
    "Camera Image" <- w265
  }
  n176 = while {
    tunnel: [w303] -> _
    tunnel: w68 -> [w302]
    tunnel: w64 -> [w301]
    tunnel: w63 -> [w300]
    tunnel: w62 -> [_]
    tunnel: w58 -> [w299]
    tunnel: w25 -> [w298]
    tunnel: w23 -> [w297]
    shift-right: [w296] -> _
    shift-left: _ -> [w295]
    tunnel: w17 -> [w294]
    i -> [w303]
    stop <- FALSE stop-if-true
    n177 = event shown="[0] Timeout" {
      selector: w300 -> [_ _ _ _ _ _ _ _ _ _ _ _ _ _ _ _ _ _ _ _ _ _]
      dyn-events: [_ _ _ _ _ _ _ _ _ _ _ _ _ _ _ _ _ w570 _ _ _ _] -> _
      timeout: u32 60 ("milliseconds to wait") -> [_ _ _ _ _ _ _ _ _ _ _ _ _ _ _ _ _ _ _ _ _ _]
      tunnel: w302 -> [w315 _ _ _ _ _ _ _ _ _ _ _ _ _ _ _ _ _ _ _ _ _]
      tunnel: "Test Tree" -> [_ _ _ _ _ _ _ _ _ _ _ _ w537 w545 w547 w551 w559 _ _ _ _ _]
      tunnel: w301 -> [_ _ _ _ _ _ _ _ _ _ _ _ _ _ _ _ _ w572 _ w590 _ _]
      tunnel: w299 -> [_ _ _ _ _ _ _ _ _ _ _ _ _ _ _ _ _ w568 _ _ _ _]
      tunnel: w298 -> [_ _ _ _ _ _ _ _ _ _ _ _ _ _ _ _ _ w566 _ _ _ _]
      tunnel: w297 -> [w310 _ _ _ _ _ _ w488 _ _ _ _ _ _ _ _ _ _ _ _ _ _]
      tunnel: [w309 w358 w460 w465 w474 w478 w482 w486 w495 w505 w512 w524 w536 w543 w546 w550 w558 w565 w585 w587 w591 w604] -> w296
      tunnel: w295 -> [w309 w358 w460 w465 w474 w478 w482 w486 _ _ w512 w524 w536 w543 w546 w550 w558 w565 w585 w587 w591 w604]
      tunnel: w294 -> [w307 _ _ _ _ _ _ _ _ _ _ _ _ _ _ _ _ _ _ _ _ _]
      event Timeout {
        n178 = event-data() -> ()  [unwired: 1 in, 1 out]
        n179 = local read "Mode"() -> (w312:T4)
        n180 = case shown="\"Test\"" "Dashboard Tab" {
          tunnel: w315 -> [_ _ w331 _ _]
          tunnel: "TestMode/Automatic/" ("Name Pattern") -> [_ _ w330 _ _]
          tunnel: T24 [{"Operation"=enum."Clear", "Color Box"=14013909}, {"Operation"=enum."Clear", "Color Box"=14013909}, {"Operation"=enum."Clear", "Color Box"=14013909}, {"Operation"=enum."Clear", "Color Box"=14013909}, {"Operation"=enum."Update", "Color Box"=14013909}, {"Operation"=enum."Update", "Color Box"=16777215}, {"Operation"=enum."Clear", "Color Box"=14013909}, {"Operation"=enum."Clear", "Color Box"=14013909}, {"Operation"=enum."Clear", "Color Box"=14013909}] -> [_ _ w323 _ w351]
          tunnel: w312 -> [_ _ w322 _ w350]
          tunnel: u32[] [15790320, 15790320, 15790320, 15790320, 16777215, 16777215, 15790320, 15790320, 15790320] -> [_ _ _ _ w356]
          tunnel: w310 -> [_ _ _ _ w344]
          tunnel: w307 -> [_ w317 _ _ _]
          frame "Auto", Default {
          }
          frame "Basic" {
            n181 = call <vilib>:"WPI_DashboardUpdateNames.vi"("Controls on Tab"=w317) -> ()  [unwired: 11 in]
          }
          frame "Test" {
            w329 = -2 ("Active Item:Row Number")
            n182 = Index Array(array=w323, index=w322) -> (element=w324:T27)
            n183 = Unbundle(w324) -> ("Operation"=w325:enum16{"Update", "Clear"}, "Color Box"=w326:u32)
            n184 = call <vilib>:"NT Read String.vi"("Name"="TestMode/TestName") -> ("String"=w320:string)  [unwired: 9 in, 1 out]
            n185 = call <vilib>:"NT Read and Format Entries as Tree.vi"("Operation"=w325, "Name Pattern"=w330, "Tree Refnum"=w331) -> ()  [unwired: 7 in, 2 out]
            n186 = case shown="\"\"" w320 {
              tunnel: "TestMode/TestProgress" ("Name") -> [w333 _]
              tunnel: "TestMode/TestProgressText" ("Name") -> [w332 _]
              frame Default {
                n187 = call <vilib>:"NT Read Number.vi"("Name"=w333) -> ("Numeric"=w334:dbl)  [unwired: 9 in, 1 out]
                n188 = call <vilib>:"NT Read String.vi"("Name"=w332) -> ("String"=w335:string)  [unwired: 9 in, 1 out]
                n189 = Bundle("Numeric"=w334, "String"=w335) -> (→"Progress":cluster{"Numeric":dbl, "String":string})  [unwired: 1 in]
              }
              frame "" {
                n190 = property on="Progress" class="Clust (strict)"("Visible"=FALSE) -> ()  [unwired: 2 in, 2 out]
                n191 = local write "Test Name"(u16 0) -> ()
              }
            }
            n192 = property on="Test Tree" class="Tree (strict)"("Active Item Row Number"=w329, "ActiveColNum"=w329, "CellBG"=w326, "Active Item Row Number"=-1 ("Active Item:Row Number"), "CellBG"=u32 5789784 ("Color Box")) -> ()  [unwired: 2 in, 2 out]
          }
          frame "Variables" {
            w341 = string[] ["CameraPublisher", "Usage", "DB"]  # Items to initially close
            n193 = First Call?() -> (First Call?: T/F=w342:bool)
            n194 = control-ref of="Tree"() -> (w343:refnum<vi>)
            n195 = Select(t=w341, s=w342, f=string[] []) -> (s? t:f=w339:string[])
            n196 = call <vilib>:"NT Read and Format Entries as Tree.vi"("Tags to  Close"=w339, "Tree Refnum"=w343) -> ()  [unwired: 8 in, 2 out]
          }
          frame "Commands" {
            w352 = u32 5789784 ("Color Box")
            w353 = T28 {"Row"=-1, "Column"=-2} ("Active Cell:Active Cell")
            w355 = T28 {"Row"=-2, "Column"=-2} ("Active Cell:Active Cell")
            n197 = Index Array(array=w356, index=w350) -> (element=w354:u32)
            n198 = Index Array(array=w351, index=w350) -> (element=w349:T27)
            n199 = Unbundle(w349) -> ("Operation"=w348:enum16{"Update", "Clear"})  [unwired: 1 out]
            n200 = local read "Command Selection"() -> (w347:i32)
            n201 = property on="Command Selection" class="MCListbox (strict)"("ActiveCell"=w355, "CellBG"=w354, "ActiveCell"=w353, "CellBG"=w352) -> ()  [unwired: 2 in, 2 out]
            n202 = call <vilib>:"WPI_DashboardUpdate RPC Info.vi"("Operation"=w348) -> ("update"=w346:bool, "commands"=w345:string[][])  [unwired: 9 in]
            n203 = property on="Command Selection" class="MCListbox (strict)"("ItemNames"=w345) -> ()  [unwired: 2 in, 2 out]
            n204 = property on="Command Params" class="Tbl (strict)"("Active Cell"=w355, "Cell BG Color"=w354, "Active Cell"=w353, "Cell BG Color"=w352) -> ()  [unwired: 2 in, 2 out]
            n205 = call <vilib>:"WPI_DashboardUpdate Command Params.vi"("Update"=w346, "NewVal"=w347, "Commands"=w345, "Param Tbl"=w344) -> ()  [unwired: 7 in, 1 out]
          }
        }
        n206 = call <vilib>:"Connextion Info.vi"() -> ("Connected"=→"NT Connection":bool)  [unwired: 10 in, 1 out]
      }
      event "Test Tree": Value Change {
        # "Show appropriate\ncontrols"
        n207 = event-data() -> ("CtlRef"=w361:refnum<vi>, "NewVal"=w359:string)  [unwired: 1 in]
        n208 = call <vilib>:"WPI_UtilitiesGetTreeIOName.vi"("NewVal"=w359, "TreeControl in"=w361) -> ("I/O Name"=w362:string)  [unwired: 9 in]
        n209 = case shown="\"Camera\"" w362 {
          selector: w362 -> [_ w369 _ w391 w400 _]
          tunnel: w359 -> [_ _ w388 w390 _ w407]
          tunnel: cluster{string[]}[] [{["640x480", "320x240", "160x120"]}, {["Auto", "Fixed indoor", "Fixed outdoor 1", "Fixed outdoor 2", "Fixed fluorescent 1", "Fixed fluorescent 2", "Hold current"]}, {["Auto", "Flicker-free 50 Hz", "Flicker-free 60 Hz", "Hold current"]}, {["None", "Prioritize frame rate", "Prioritize image quality"]}, {["Monochrome", "Color"]}] -> [_ _ _ _ _ w406]
          frame Default {
            w364 = FALSE ("Visible")
            w363 = FALSE ("Visible")
            n210 = property on="Motor" class="Clust (strict)"("Visible"=w363) -> ()  [unwired: 2 in, 2 out]
            n211 = property on="Test Ring" class="Ring (strict)"("Visible"=w363) -> ()  [unwired: 2 in, 2 out]
            n212 = property on="Rev/Fwd" class="Clust (strict)"("Visible"=w364) -> ()  [unwired: 2 in, 2 out]
            n213 = property on="On/Off" class="Bool (strict)"("Visible"=w364) -> ()  [unwired: 2 in, 2 out]
            n214 = property on="Test Slider" class="Slide (strict)"("Visible"=w364) -> ()  [unwired: 2 in, 2 out]
          }
          frame "Analog Out", "Motor", "PWM" {
            w370 = FALSE ("Visible")
            n215 = case shown="\"Analog Out\"" w369 {
              tunnel: [1.0 ("Value") -1.0 ("Value") 0.0 ("Value")] -> w368
              tunnel: [255.0 ("Value") 1.0 ("Value") 5.0 ("Value")] -> w367
              tunnel: [128.0 ("Value") 0.0 ("Value") 0.0 ("Value")] -> w366
              tunnel: [64.0 ("Value") 0.5 ("Value") 1.0 ("Value")] -> w365
              frame "PWM" {
              }
              frame "Motor", Default {
              }
              frame "Analog Out" {
              }
            }
            n216 = property on="Motor" class="Clust (strict)"("Visible"=TRUE) -> ()  [unwired: 2 in, 2 out]
            n217 = property on="Value" class="Slide (strict)"("Value"=w366, "Scale.Minimum"=w368, "Scale.Maximum"=w367, "Scale.Increment"=w365) -> ()  [unwired: 2 in, 2 out]
            n218 = property on="On/Off" class="Bool (strict)"("Visible"=w370) -> ()  [unwired: 2 in, 2 out]
            n219 = property on="Test Slider" class="Slide (strict)"("Visible"=w370) -> ()  [unwired: 2 in, 2 out]
            n220 = property on="Test Ring" class="Ring (strict)"("Visible"=w370) -> ()  [unwired: 2 in, 2 out]
            n221 = property on="Rev/Fwd" class="Clust (strict)"("Visible"=w370) -> ()  [unwired: 2 in, 2 out]
          }
          frame "Servo" {
            w386 = FALSE ("Visible")
            n222 = call <vilib>:"NT Read Number.vi"("Name"=w388) -> ("Numeric"=w387:dbl)  [unwired: 9 in, 1 out]
            n223 = property on="Test Slider" class="Slide (strict)"("Visible"=TRUE, "Scale.Maximum"=170.0 ("Scale.Range:Maximum")) -> ()  [unwired: 2 in, 2 out]
            n224 = local write "Test Slider"(w387) -> ()
            n225 = property on="Motor" class="Clust (strict)"("Visible"=w386) -> ()  [unwired: 2 in, 2 out]
            n226 = property on="Rev/Fwd" class="Clust (strict)"("Visible"=w386) -> ()  [unwired: 2 in, 2 out]
            n227 = property on="On/Off" class="Bool (strict)"("Visible"=w386) -> ()  [unwired: 2 in, 2 out]
            n228 = property on="Test Ring" class="Ring (strict)"("Visible"=w386) -> ()  [unwired: 2 in, 2 out]
          }
          frame "Relay", "Solenoid" {
            w389 = FALSE ("Visible")
            n229 = property on="Motor" class="Clust (strict)"("Visible"=w389) -> ()  [unwired: 2 in, 2 out]
            n230 = property on="Test Slider" class="Slide (strict)"("Visible"=w389) -> ()  [unwired: 2 in, 2 out]
            n231 = Search and Replace String(input string=w390, search string="/Value  **", replace string="/Direction") -> (result string=w396:string)  [unwired: 5 in, 3 out]
            n232 = property on="Test Ring" class="Ring (strict)"("Visible"=w389) -> ()  [unwired: 2 in, 2 out]
            n233 = call <vilib>:"NT Read String.vi"("Name"=w396) -> ("String"=w394:string)  [unwired: 9 in, 1 out]
            n234 = Equal?(x="Both directions", y=w394) -> (x = y?=w392:bool)
            n235 = Not(x=w392) -> (.not. x?=w393:bool)
            n236 = property on="Rev/Fwd" class="Clust (strict)"("Visible"=w392) -> ()  [unwired: 2 in, 2 out]
            n237 = property on="On/Off" class="Bool (strict)"("Visible"=w393, "Caption.Text"=w391) -> ()  [unwired: 2 in, 2 out]
          }
          frame "Compressor", "Digital Out" {
            w399 = FALSE ("Visible")
            # "Get direction and finish"
            n238 = property on="Motor" class="Clust (strict)"("Visible"=w399) -> ()  [unwired: 2 in, 2 out]
            n239 = property on="Test Slider" class="Slide (strict)"("Visible"=w399) -> ()  [unwired: 2 in, 2 out]
            n240 = property on="Test Ring" class="Ring (strict)"("Visible"=w399) -> ()  [unwired: 2 in, 2 out]
            n241 = property on="On/Off" class="Bool (strict)"("Visible"=TRUE, "Caption.Text"=w400) -> ()  [unwired: 2 in, 2 out]
            n242 = property on="Rev/Fwd" class="Clust (strict)"("Visible"=FALSE) -> ()  [unwired: 2 in, 2 out]
          }
          frame "Camera" {
            n243 = call <vilib>:"Get Last Path Segment.vi"("String in"=w407) -> ("String out"=w408:string)  [unwired: 10 in]
            n244 = property on="On/Off" class="Bool (strict)"("Visible"=FALSE) -> ()  [unwired: 2 in, 2 out]
            n245 = property on="Motor" class="Clust (strict)"("Visible"=FALSE) -> ()  [unwired: 2 in, 2 out]
            n246 = property on="Rev/Fwd" class="Clust (strict)"("Visible"=FALSE) -> ()  [unwired: 2 in, 2 out]
            n247 = case shown="\"White Balance  **\"" w408 {
              tunnel: w407 -> [w414 w423 w432 w441 w450 _ w456]
              tunnel: w406 -> [w412 w420 w429 w438 w447 _ _]
              frame "Size  **" {
                n248 = Index Array(array=w412) -> (element=w411:cluster{string[]})  [unwired: 1 in]
                n249 = call <vilib>:"NT Read String.vi"("Name"=w414) -> ("String"=w413:string)  [unwired: 9 in, 1 out]
                n250 = Unbundle(w411) -> (w409:string[])
                n251 = Match First String(2:w409, 3:w413) -> (0:w410:i32)  [unwired: 1 out]
                n252 = property on="Test Ring" class="Ring (strict)"("Value"=w410, "Strings []"=w409) -> ()  [unwired: 2 in, 2 out]
                n253 = property on="Test Ring" class="Ring (strict)"("Visible"=TRUE) -> ()  [unwired: 2 in, 2 out]
                n254 = property on="Test Slider" class="Slide (strict)"("Visible"=FALSE) -> ()  [unwired: 2 in, 2 out]
              }
              frame "White Balance  **" {
                n255 = Index Array(array=w420, index=1) -> (element=w421:cluster{string[]})
                n256 = call <vilib>:"NT Read String.vi"("Name"=w423) -> ("String"=w422:string)  [unwired: 9 in, 1 out]
                n257 = Unbundle(w421) -> (w418:string[])
                n258 = Match First String(2:w418, 3:w422) -> (0:w417:i32)  [unwired: 1 out]
                n259 = property on="Test Ring" class="Ring (strict)"("Value"=w417, "Strings []"=w418) -> ()  [unwired: 2 in, 2 out]
                n260 = property on="Test Ring" class="Ring (strict)"("Visible"=TRUE) -> ()  [unwired: 2 in, 2 out]
                n261 = property on="Test Slider" class="Slide (strict)"("Visible"=FALSE) -> ()  [unwired: 2 in, 2 out]
              }
              frame "Exposure  **" {
                n262 = Index Array(array=w429, index=2) -> (element=w430:cluster{string[]})
                n263 = call <vilib>:"NT Read String.vi"("Name"=w432) -> ("String"=w431:string)  [unwired: 9 in, 1 out]
                n264 = Unbundle(w430) -> (w426:string[])
                n265 = Match First String(2:w426, 3:w431) -> (0:w427:i32)  [unwired: 1 out]
                n266 = property on="Test Ring" class="Ring (strict)"("Value"=w427, "Strings []"=w426) -> ()  [unwired: 2 in, 2 out]
                n267 = property on="Test Ring" class="Ring (strict)"("Visible"=TRUE) -> ()  [unwired: 2 in, 2 out]
                n268 = property on="Test Slider" class="Slide (strict)"("Visible"=FALSE) -> ()  [unwired: 2 in, 2 out]
              }
              frame "Exposure Priority  **" {
                n269 = Index Array(array=w438, index=3) -> (element=w439:cluster{string[]})
                n270 = call <vilib>:"NT Read String.vi"("Name"=w441) -> ("String"=w440:string)  [unwired: 9 in, 1 out]
                n271 = Unbundle(w439) -> (w435:string[])
                n272 = Match First String(2:w435, 3:w440) -> (0:w436:i32)  [unwired: 1 out]
                n273 = property on="Test Ring" class="Ring (strict)"("Value"=w436, "Strings []"=w435) -> ()  [unwired: 2 in, 2 out]
                n274 = property on="Test Ring" class="Ring (strict)"("Visible"=TRUE) -> ()  [unwired: 2 in, 2 out]
                n275 = property on="Test Slider" class="Slide (strict)"("Visible"=FALSE) -> ()  [unwired: 2 in, 2 out]
              }
              frame "Color Enable  **" {
                n276 = Index Array(array=w447, index=4) -> (element=w448:cluster{string[]})
                n277 = call <vilib>:"NT Read String.vi"("Name"=w450) -> ("String"=w449:string)  [unwired: 9 in, 1 out]
                n278 = Unbundle(w448) -> (w444:string[])
                n279 = Match First String(2:w444, 3:w449) -> (0:w445:i32)  [unwired: 1 out]
                n280 = property on="Test Ring" class="Ring (strict)"("Value"=w445, "Strings []"=w444) -> ()  [unwired: 2 in, 2 out]
                n281 = property on="Test Ring" class="Ring (strict)"("Visible"=TRUE) -> ()  [unwired: 2 in, 2 out]
                n282 = property on="Test Slider" class="Slide (strict)"("Visible"=FALSE) -> ()  [unwired: 2 in, 2 out]
              }
              frame Default {
                n283 = property on="Test Ring" class="Ring (strict)"("Visible"=FALSE) -> ()  [unwired: 2 in, 2 out]
                n284 = property on="Test Slider" class="Slide (strict)"("Visible"=FALSE) -> ()  [unwired: 2 in, 2 out]
              }
              frame "Brightness  **", "Color Level  **", "Compression  **", "FPS  **", "Sharpness  **" {
                n285 = call <vilib>:"NT Read Number.vi"("Name"=w456) -> ("Numeric"=w455:dbl)  [unwired: 9 in, 1 out]
                n286 = local write "Test Slider"(w455) -> ()
                n287 = property on="Test Slider" class="Slide (strict)"("Visible"=TRUE, "Scale.Maximum"=100.0 ("Scale.Range:Maximum")) -> ()  [unwired: 2 in, 2 out]
                n288 = property on="Test Ring" class="Ring (strict)"("Visible"=FALSE) -> ()  [unwired: 2 in, 2 out]
              }
            }
          }
        }
        n289 = property on="Progress" class="Clust (strict)"("Visible"=FALSE) -> ()  [unwired: 2 in, 2 out]
      }
      event "Test Name": Mouse Enter {
        # "Populate the ring with the list of tests"
        n290 = event-data() -> ()  [unwired: 1 in, 1 out]
        n291 = call <vilib>:"NT Read String Array.vi"("Name"="TestMode/TestList") -> ("String Array"=w464:string[])  [unwired: 9 in, 1 out]
        n292 = Build Array (concatenate)("Select the test to run...", w464) -> (w463:string[])
        n293 = property on="Test Name" class="Ring (strict)"("Strings []"=w463) -> ()  [unwired: 2 in, 2 out]
      }
      event "Test Name": Value Change {
        w466 = FALSE ("Visible")
        # "Tell the robot the test name to run"
        n294 = event-data() -> ("NewVal"=w470:u16)  [unwired: 1 in]
        n295 = property on="Test Name" class="Ring (strict)"() -> ("Strings []"=w471:string[])  [unwired: 2 in, 2 out]
        n296 = local write "Progress"(T6 {"Test Progress"=0, "Test Progress Text"=""} ("Progress")) -> ()
        n297 = Index Array(array=w471, index=w470) -> (element=w469:string)
        n298 = call <vilib>:"NT Write String.vi"("String"=w469, "Name"="TestMode/TestName") -> ()  [unwired: 9 in, 1 out]
        n299 = property on="Progress" class="Clust (strict)"("Visible"=TRUE) -> ()  [unwired: 2 in, 2 out]
        n300 = property on="Motor" class="Clust (strict)"("Visible"=w466) -> ()  [unwired: 2 in, 2 out]
        n301 = property on="Test Slider" class="Slide (strict)"("Visible"=w466) -> ()  [unwired: 2 in, 2 out]
        n302 = property on="On/Off" class="Bool (strict)"("Visible"=w466) -> ()  [unwired: 2 in, 2 out]
        n303 = property on="Rev/Fwd" class="Clust (strict)"("Visible"=w466) -> ()  [unwired: 2 in, 2 out]
        n304 = property on="Test Ring" class="Ring (strict)"("Visible"=w466) -> ()  [unwired: 2 in, 2 out]
      }
      event "Select Auto": Mouse Enter {
        # "Populate the combo box with the list of autonomous options"
        n305 = event-data() -> ()  [unwired: 1 in, 1 out]
        n306 = call <vilib>:"NT Read String Array.vi"("Name"="Auto List") -> ("String Array"=w473:string[])  [unwired: 9 in, 1 out]
        n307 = property on="Select Auto" class="CmbBox"("Strings[]"=w473) -> ()  [unwired: 2 in, 2 out]
      }
      event "Select Auto": Value Change {
        # "User modified the Auto Selection. Write to NT variable so robot knows."
        n308 = event-data() -> ("NewVal"=w476:string)  [unwired: 1 in]
        n309 = call <vilib>:"NT Write String.vi"("String"=w476, "Name"="Auto Selector") -> ()  [unwired: 9 in, 1 out]
      }
      event "Select Robot Position": Value Change {
        n310 = event-data() -> ("NewVal"=w480:string)  [unwired: 1 in, 5 out]
        n311 = case shown="\"Left\", Default" w480 {
          tunnel: [0 i8 1 i8 2] -> w479
          frame "Left", Default {
          }
          frame "Right" {
          }
          frame "Center" {
          }
        }
        n312 = call <vilib>:"NT Write String.vi"("String"=w480, "Name"="Robot Position") -> ()  [unwired: 9 in, 1 out]
        n313 = property on="Ring" class="Ring (strict)"("Val(Sgnl)"=w479) -> ()  [unwired: 2 in, 2 out]
      }
      event "Command Selection": Value Change {
        # "Get the params and show in table"
        n314 = event-data() -> ("NewVal"=w489:i32)  [unwired: 1 in]
        n315 = property on="Command Selection" class="MCListbox (strict)"() -> ("ItemNames"=w487:string[][])  [unwired: 2 in, 2 out]
        n316 = call <vilib>:"WPI_DashboardUpdate Command Params.vi"("NewVal"=w489, "Commands"=w487, "Param Tbl"=w488) -> ()  [unwired: 8 in, 1 out]
      }
      event "Execute Command": Value Change {
        # "Started one, Unique ID holds\nresponse"
        n317 = event-data() -> ()  [unwired: 1 in, 1 out]
        n318 = property on="Command Selection" class="MCListbox (strict)"() -> ("ItemNames"=w500:string[][])  [unwired: 2 in, 2 out]
        n319 = Index Array(array=w500, index (row)="Command Selection", index (col)=0) -> (element=w498:string)
        n320 = call <vilib>:"Invoke Commands.vi"("Command Params"="Command Params", "Function Name"=w498) -> ("Params"=w494:u8, "Started"=w493:bool)  [unwired: 7 in, 1 out]
        n321 = Array Subset(array="Command Params", length (row)=w494) -> (w495:string[][])  [unwired: 3 in]
        n322 = Select(t="Executing" ("Cmd Status"), s=w493, f="" ("Cmd Status")) -> (s? t:f=→"Cmd Status":string)
      }
      event "Command Selection": Double Click {
        n323 = event-data() -> ("Row"=w508:i32)  [unwired: 1 in]
        n324 = property on="Command Selection" class="MCListbox (strict)"() -> ("ItemNames"=w511:string[][])  [unwired: 2 in, 2 out]
        n325 = local read "Command Params"() -> (w507:string[][])
        n326 = Index Array(array=w511, index (row)=w508, index (col)=0) -> (element=w509:string)
        n327 = call <vilib>:"Invoke Commands.vi"("Command Params"=w507, "Function Name"=w509) -> ("Params"=w506:u8, "Started"=w501:bool)  [unwired: 7 in, 1 out]
        n328 = Array Subset(array=w507, length (row)=w506) -> (w505:string[][])  [unwired: 3 in]
        n329 = Select(t="Executing" ("Cmd Status"), s=w501, f="" ("Cmd Status")) -> (s? t:f=w502:string)
        n330 = local write "Cmd Status"(w502) -> ()
      }
      event "CheckList": Double Click {
        # "Shift clears all"
        # "Update symbols on the listbox"
        n331 = event-data() -> ("PlatMods.Shift"=w513:bool, "Row"=w515:i32)  [unwired: 1 in]
        n332 = case shown="True" w513 {
          tunnel: w515 -> [w519 _]
          tunnel: 1 -> [w518 _]
          frame False {
            n333 = property on="CheckList" class="LstBox (strict)"() -> ("Item Symbols"=w517:i32[])  [unwired: 2 in, 2 out]
            n334 = Replace Array Subset(array=w517, new element=w518, index=w519) -> (w516:i32[])
            n335 = property on="CheckList" class="LstBox (strict)"("Item Symbols"=w516) -> ()  [unwired: 2 in, 2 out]
          }
          frame True {
            w520 = 0 ("Top Row")
            n336 = property on="CheckList" class="LstBox (strict)"() -> ("Number of Rows"=w522:u32)  [unwired: 2 in, 2 out]
            n337 = Initialize Array(0, w522) -> (w521:i32[])
            n338 = property on="CheckList" class="LstBox (strict)"("Top Row"=w520, "Value"=w520, "Item Symbols"=w521) -> ()  [unwired: 2 in, 2 out]
          }
        }
      }
      event "CheckList": Key Down {
        # "Update symbols on the listbox\nLeft and right keys check and uncheck"
        n339 = event-data() -> ("VKey"=w526:T25)  [unwired: 1 in]
        n340 = case shown="\"Left\", \"Right\"" w526 {
          selector: w526 -> [w531 _]
          tunnel: eventvkey."Left" ("VKey") -> [w529 _]
          frame "Left", "Right" {
            n341 = Equal?(x=w529, y=w531) -> (x = y?=w530:bool)
            n342 = Select(t=0, s=w530, f=1) -> (s? t:f=w532:i32)
            n343 = property on="CheckList" class="LstBox (strict)"() -> ("Item Symbols"=w535:i32[])  [unwired: 2 in, 2 out]
            n344 = Replace Array Subset(array=w535, new element=w532, index="CheckList") -> (w534:i32[])
            n345 = property on="CheckList" class="LstBox (strict)"("Item Symbols"=w534) -> ()  [unwired: 2 in, 2 out]
          }
          frame Default {
          }
        }
      }
      event "Motor.Enable": Value Change {
        # "When the test mode otor enable helper is set, update that\ntree row item's value"
        n346 = event-data() -> ("NewVal"=w541:bool)  [unwired: 1 in]
        n347 = Unbundle("Motor") -> ("Value"=w540:dbl)  [unwired: 1 out]
        n348 = Select(t=w540, s=w541, f=0.0) -> (s? t:f=w538:dbl)
        n349 = call <vilib>:"NT Write Number.vi"("Numeric"=w538, "Name"=w537) -> ()  [unwired: 9 in, 1 out]
      }
      event "Test Slider": Value Change {
        # "When the test mode slider helper is set, update that\ntree row item's value"
        n350 = event-data() -> ("NewVal"=w544:dbl)  [unwired: 1 in]
        n351 = call <vilib>:"NT Write Number.vi"("Numeric"=w544, "Name"=w545) -> ()  [unwired: 9 in, 1 out]
      }
      event "On/Off": Value Change {
        # "When the test mode on/off helper value is set, update that\ntree row item's value"
        n352 = event-data() -> ("NewVal"=w549:bool)  [unwired: 1 in]
        n353 = Boolean To (0,1)(Boolean=w549) -> (0, 1=w548:i16)
        n354 = call <vilib>:"NT Write Number.vi"("Numeric"=w548, "Name"=w547) -> ()  [unwired: 9 in, 1 out]
      }
      event "Rev/Fwd": Value Change {
        # "When the test mode helper value for relays is set, update that\ntree row item's value"
        n355 = event-data() -> ("NewVal.Forward"=w557:bool, "NewVal.Reverse"=w556:bool)  [unwired: 1 in]
        n356 = Boolean To (0,1)(Boolean=w557) -> (0, 1=w553:i16)
        n357 = Boolean To (0,1)(Boolean=w556) -> (0, 1=w555:i16)
        n358 = Negate(x=w555) -> (-x=w554:i16)
        n359 = Add(x=w553, y=w554) -> (x+y=w552:i16)
        n360 = call <vilib>:"NT Write Number.vi"("Numeric"=w552, "Name"=w551) -> ()  [unwired: 9 in, 1 out]
      }
      event "Test Ring": Value Change {
        # "When a test mode helper value is selected from the ring,\nset the tree item's variable to the string value"
        n361 = event-data() -> ("NewVal"=w561:u16)  [unwired: 1 in]
        n362 = property on="Test Ring" class="Ring (strict)"() -> ("Strings []"=w562:string[])  [unwired: 2 in, 2 out]
        n363 = Index Array(array=w562, index=w561) -> (element=w560:string)
        n364 = call <vilib>:"NT Write String.vi"("String"=w560, "Name"=w559) -> ()  [unwired: 9 in, 1 out]
      }
      event "Rec Mode": Value Change {
        # "Update globals for recording mode and path to read log from.\nClear when logging and let NetworkTables set path for vision to\nuse."
        n365 = event-data() -> ("NewVal"=w573:enum32{"Stop", "Record", "Playback"})  [unwired: 1 in]
        n366 = global write "WPI_DashboardLogging Global.vi" "Logging Filename"(path "") -> ()
        n367 = global write "WPI_DashboardLogging Global.vi" "Recording"(w573) -> ()
        n368 = case shown="\"Playback\"" w573 {
          tunnel: w572 -> [_ w575 w584]
          tunnel: [_ _ w583] -> w570
          tunnel: [_ _ w582] -> _
          tunnel: w568 -> [_ _ w580]
          tunnel: cluster{i32, i32} {-250, 170} -> [_ _ w579]
          tunnel: [_ _ T26 {"Image Size"=TRUE, "Image Type"=TRUE, "Pixel Value"=TRUE, "ROI Information"=TRUE, "Zoom Factor"=FALSE} ("Image Information Shown:All Elements")] -> w563
          tunnel: [_ _ TRUE ("Zoom Factor")] -> w564
          tunnel: w566 -> [_ _ w576]
          frame Default {
          }
          frame "Stop", "Record" {
            # "Place Window too"
            n369 = invoke class="VI" method="FP.Close"(reference=w575) -> (reference out=w574:refnum<vi>)  [unwired: 2 in, 2 out]
            n370 = invoke class="VI" method="Abort VI"(reference=w574) -> ()  [unwired: 2 in, 3 out]
          }
          frame "Playback" {
            n371 = call "Open Playback Panel.vi"("Offset"=w579, "DB VI Ref"=w580, "Playback in"=w584) -> ("Playback out"=w581:refnum<vi>)  [unwired: 8 in]
            n372 = register-events(w581, w576) -> (reference out=w583:refnum<event-registration>, error out=w582:errorcluster)  [unwired: 2 in]
          }
        }
        n373 = property on="Camera Image Right" class="ImageControl"("Image Information Shown"=w563, "Image Information Visible"=w564) -> ()  [unwired: 2 in, 2 out]
        n374 = property on="Camera Image" class="ImageControl"("Image Information Shown"=w563, "Image Information Visible"=w564) -> ()  [unwired: 2 in, 2 out]
        n375 = call <vilib>:"WPI_DashboardNT Log FieldName Cache.vi"("Operation"=enum16{"Lookup/Add", "Index", "Clear"}."Clear") -> ()  [unwired: 8 in, 3 out]
      }
      event Panel Close {
        w586 = enum32{"Stop", "Record", "Playback"}."Stop" ("Rec Mode")
        # "Playback window has been closed, abort"
        n376 = event-data() -> ()  [unwired: 1 in, 4 out]
        n377 = local write "Rec Mode"(w586) -> ()
        n378 = global write "WPI_DashboardLogging Global.vi" "Recording"(w586) -> ()
      }
      event Panel Close {
        # "Abort playback window and ourself"
        n379 = event-data() -> ()  [unwired: 1 in, 4 out]
        n380 = invoke class="VI" method="FP.Close"(reference=w590) -> (reference out=w589:refnum<vi>)  [unwired: 2 in, 2 out]
        n381 = invoke class="VI" method="Abort VI"(reference=w589) -> (error out=w588:errorcluster)  [unwired: 2 in, 2 out]
        n382 = invoke class="VI" method="Abort VI"(error in=w588) -> ()  [unwired: 2 in, 3 out]
      }
      event User Event {
        n383 = event-data() -> ("IDs"=w597:cluster{"RPC field ID":u16, "Unique ID":u16}, "String"=w596:string)  [unwired: 1 in]
        n384 = Bundle("IDs"=w597, "String"=w596) -> (w595:T11)  [unwired: 1 in]
        n385 = call <vilib>:"Retrieve RPC Response.vi"("RPC Response"=w595) -> ("Output"=w593:string[][])  [unwired: 10 in]
        n386 = Build Array (concatenate)(w591, w593) -> (w592:string[][])
        n387 = local write "Command Params"(w592) -> ()
        n388 = local write "Cmd Status"("" ("Cmd Status")) -> ()
      }
      event "Tree": Double Click {
        n389 = event-data() -> ("PlatMods"=w603:T29, "Tag"=w600:string)  [unwired: 1 in]
        n390 = Unbundle(w603) -> ("Shift"=w602:bool)  [unwired: 4 out]
        n391 = String Subset(string=w600, length (rest)=1 ("length (rest)")) -> (substring=w599:string)  [unwired: 1 in]
        n392 = Not(x=w602) -> (.not. x?=w601:bool)
        n393 = case shown="\"/\"" w599 {
          tunnel: w600 -> [_ w606]
          tunnel: w601 -> [_ w605]
          frame Default {
          }
          frame "/" {
            n394 = call <vilib>:"NT Update Persistence.vi"("Persistence"=w605, "Name"=w606) -> ()  [unwired: 9 in, 1 out]
          }
        }
      }
    }
  }
  n395 = while {
    tunnel: w65 -> [w608]
    i -> [w611]
    stop <- FALSE stop-if-true
    n396 = Wait (ms)(milliseconds to wait=u32 100) -> ()  [unwired: 1 out]
    n397 = case shown="\"Playback\"" "Rec Mode" {
      tunnel: w611 -> [_ _ w626]
      tunnel: [u32 2829099 ("Base Color") u32 11141120 ("Target Color") w615] -> w607
      frame "Stop", Default {
        # "Reset the color, extra updates don't cost much"
      }
      frame "Record" {
      }
      frame "Playback" {
        # "Playback"
        n398 = Quotient & Remainder(x=w626, y=u32 50 ("milliseconds to wait")) -> (x-y*floor(x/y)=w622:u32)  [unwired: 1 out]
        n399 = Divide(x=w622, y=u32 50 ("milliseconds to wait")) -> (x/y=w619:dbl)
        n400 = Multiply(x=6.283185307179586, y=w619) -> (x*y=w624:dbl)
        n401 = Sine(x=w624) -> (sin(x)=w623:dbl)
        n402 = Absolute Value(x=w623) -> (abs(x)=w616:dbl)
        n403 = call "Interpolate RGB Color.vi"("Proportion"=w616, "Target Color"=u32 30976, "Base Color"=u32 2829099) -> ("Result Color"=w615:u32)  [unwired: 8 in]
      }
    }
    n404 = property class="Pane"(reference=w608, "PaneColor"=w607) -> ()  [unwired: 1 in, 2 out]
  }
  n405 = local write "Dashboard Tab"(T12."Auto" ("Dashboard Tab")) -> ()
  n406 = property on="On/Off" class="Bool (strict)"("Visible"=w36) -> ()  [unwired: 2 in, 2 out]
  n407 = property on="Motor" class="Clust (strict)"("Visible"=w36) -> ()  [unwired: 2 in, 2 out]
  n408 = property on="Progress" class="Clust (strict)"("Visible"=w36) -> ()  [unwired: 2 in, 2 out]
  n409 = property on="Test Ring" class="Ring (strict)"("Visible"=w36) -> ()  [unwired: 2 in, 2 out]
  n410 = property on="Rev/Fwd" class="Clust (strict)"("Visible"=w36) -> ()  [unwired: 2 in, 2 out]
  n411 = local write "Command Selection"(u16 0 ("milliseconds to wait")) -> ()
  n412 = while {
    tunnel: u16 1741 ("timeout ms (25000)") -> [w628]
    stop <- FALSE stop-if-true
    n413 = TCP Create Listener(10:w628) -> (0:w627:errorcluster, 3:w629:refnum<k5>)  [unwired: 4 in, 1 out]
    n414 = case shown="No Error" w627 {
      selector: w627 -> [w631 _]
      tunnel: w629 -> [w632 _]
      frame No Error {
        n415 = while {
          tunnel: w632 -> [w635]
          tunnel: w631 -> [w634]
          stop <- FALSE stop-if-true
          n416 = TCP Wait On Listener(8:w634, 11:w635) -> (0:w636:errorcluster, 4:w637:refnum<k5>)  [unwired: 2 in, 3 out]
          n417 = local write "TCP"(w637) -> ()
          n418 = case shown="No Error" w636 {
            frame No Error {
            }
            frame Error {
              n419 = Wait (ms)(milliseconds to wait=u32 1000) -> ()  [unwired: 1 out]
            }
          }
        }
      }
      frame Error {
        n420 = Wait (ms)(milliseconds to wait=u32 1000) -> ()  [unwired: 1 out]
      }
    }
  }
  n421 = disable-structure shown="Disabled" {
    frame Disabled {
    }
    frame Enabled {
    }
  }
  n422 = local write "Command Params"(string[][] [] ("Command Params")) -> ()
  n423 = global write "WPI_DashboardLogging Global.vi" "Recording"(w59) -> ()
  n424 = local write "Rec Mode"(w59) -> ()
  n425 = call <vilib>:"NT Write String.vi"("String"="Select Auto", "Name"="Auto Selector") -> ()  [unwired: 9 in, 1 out]
